vi "UniversalCable.vi"(7 "Cable Network Parameters":T2, 8 "Unused Output (FE/t)":ext, 11 "Push Input (FE/t)":ext) -> (0 "Output (FE/t)":ext, 3 "Rejected Input (FE/t)":ext, 4 "Buffer Size (FE)":ext, 5 "Buffered (FE)":ext)   [LabVIEW 2023]
uses:
  Tier.ctl
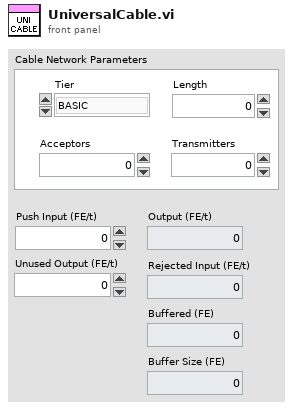
[diagram p1: front panel]
types:
  T1 = typedef "Tier.ctl" = enum16{"BASIC", "ADVANCED", "ELITE", "ULTIMATE"}
  T2 = cluster{"Tier":T1, "Acceptors":i64, "Length":i64, "Transmitters":i64}
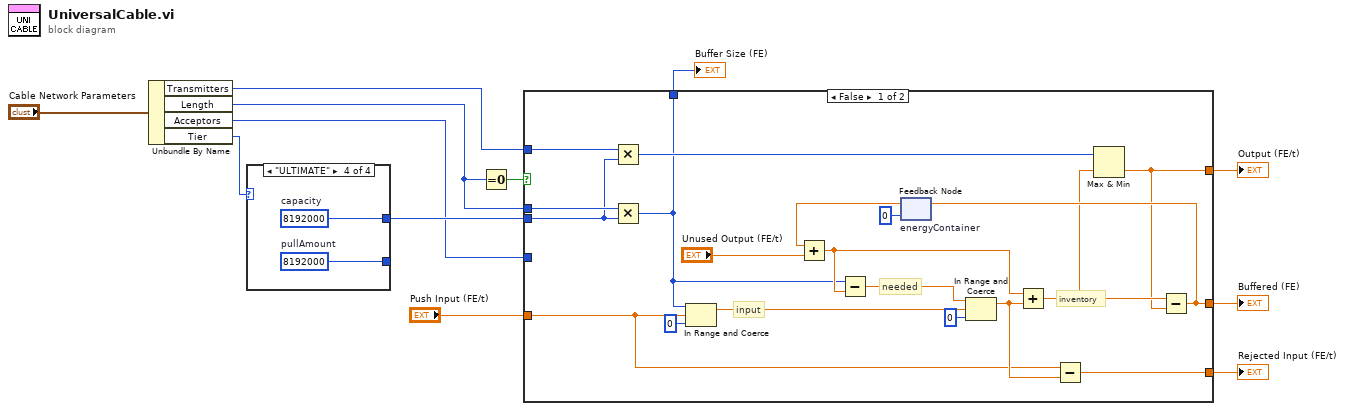
[diagram p0: block diagram]
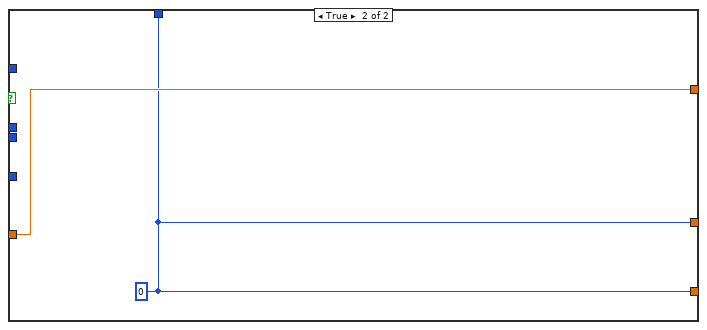
[diagram p2: hidden frame]
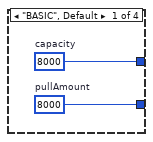
[diagram p3: hidden frame]
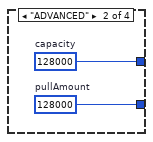
[diagram p4: hidden frame]
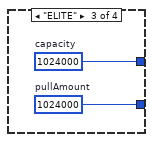
[diagram p5: hidden frame]
diagram:
  n1 = Unbundle By Name("Cable Network Parameters") -> ("Transmitters"=w1:i64, "Length"=w3:i64, "Acceptors"=w2:i64, "Tier"=w4:T1)
  n2 = case shown="\"ULTIMATE\"" w4 {
    tunnel: [w14 w16 w18 w20] -> w11
    tunnel: [w13 w15 w17 w19] -> _
    frame "BASIC", Default {
      w13 = i64 8000  # pullAmount
      w14 = i64 8000  # capacity
    }
    frame "ADVANCED" {
      w15 = i64 128000  # pullAmount
      w16 = i64 128000  # capacity
    }
    frame "ELITE" {
      w17 = i64 1024000  # pullAmount
      w18 = i64 1024000  # capacity
    }
    frame "ULTIMATE" {
      w19 = i64 8192000  # pullAmount
      w20 = i64 8192000  # capacity
    }
  }
  n3 = Equal To 0?(x=w3) -> (x = 0?=w7:bool)
  n4 = case shown="False" w7 {
    tunnel: w3 -> [w38 _]
    tunnel: [w36 w40] -> w12
    tunnel: w11 -> [w22 _]
    tunnel: [w21 w40] -> w10
    tunnel: [w39 w40] -> w9
    tunnel: [w26 w41] -> w8
    tunnel: "Push Input (FE/t)" -> [w24 w41]
    tunnel: w2 -> [_ _]
    tunnel: w1 -> [w23 _]
    frame False {
      # "inventory"
      # "needed"
      # "input"
      n5 = Multiply(x=w23, y=w22) -> (x*y=w28:i64)
      n6 = Multiply(x=w38, y=w22) -> (x*y=w21:i64)
      n7 = In Range and Coerce(upper limit=w21, x=w24, lower limit=i64 0) -> (coerced(x)=w37:ext)  [unwired: 1 out]
      n8 = feedback #1 "energyContainer"(i64 0) -> (w35:ext)
      n9 = Add(x=w35, y="Unused Output (FE/t)") -> (x+y=w30:ext)
      n10 = Subtract(x=w21, y=w30) -> (x-y=w32:ext)
      n11 = In Range and Coerce(upper limit=w32, x=w37, lower limit=i64 0) -> (coerced(x)=w29:ext)  [unwired: 1 out]
      n12 = Add(x=w30, y=w29) -> (x+y=w27:ext)
      n13 = Subtract(x=w24, y=w29) -> (x-y=w36:ext)
      n14 = Max & Min(x=w28, y=w27) -> (min(x,y)=w26:ext)  [unwired: 1 out]
      n15 = Subtract(x=w27, y=w26) -> (x-y=w39:ext)
      n16 = feedback-in #1(w39) -> ()
    }
    frame True {
      w40 = i64 0
    }
  }
  "Rejected Input (FE/t)" <- w12
  "Buffer Size (FE)" <- w10
  "Output (FE/t)" <- w8
  "Buffered (FE)" <- w9
